vi "Add.vi"(8 "error in":errorcluster, 9 "configuration version":cluster{"major":u32, "minor":u32, "fix":u32}={"major"=1, "minor"=0, "fix"=0}, 10 "framework configuration":T1, 11 "target in":refnum<k24>) -> (0 "error out":errorcluster, 2 "data sharing framework custom device":T17 format="%.0x", 3 "target out":refnum<k24>)   [LabVIEW 2017, in "Data Sharing Framework Custom Device Scripting.lvlib"]
uses:
  Data Sharing Framework Custom Device Scripting.lvlib
  NationalInstruments.VeriStand.SystemDefinitionAPI
  <vilib>/NI Veristand/Custom Device API/Custom Device Item Ref.ctl
  DSF Core.lvlibp/Typedefs/DSF Engine Framework Configuration.ctl
  DSF Core.lvlibp/Typedefs/DSF Engine Plugin Configuration.ctl
  DSF Core.lvlibp/Typedefs/Core Plugin Configuration.ctl
  DSF Core.lvlibp/Typedefs/DSF Timing Info.ctl
  DSF Core.lvlibp/Typedefs/DSF Settings Info.ctl
  DSF Core.lvlibp/Typedefs/DSF Engine Plugin Thread Configuration.ctl
  DSF Core.lvlibp/Typedefs/Core Thread Configuration.ctl
  DSF Core.lvlibp/Typedefs/DSF Engine Transfer Group Configuration.ctl
  DSF Core.lvlibp/Typedefs/Core Group Configuration.ctl
  DSF Core.lvlibp/Typedefs/DSF Direction.ctl
  DSF Core.lvlibp/Typedefs/DSF Timeout Behavior.ctl
  DSF Core.lvlibp/Typedefs/DSF Engine Transfer Configuration.ctl
  DSF Core.lvlibp/Typedefs/Core Transfer Configuration.ctl
  DSF Core.lvlibp/Typedefs/DSF Engine Channel Configuration.ctl
  DSF Core.lvlibp/Typedefs/Core Channel Configuration.ctl
  DSF Core.lvlibp/Typedefs/DSF Data Type.ctl
  Shared/DSF Shared.lvlib
  System Explorer/DSF System Explorer.lvlib
  <vilib>/NI VeriStand/Custom Device API/Custom Device API.lvlib
  DSF Core.lvlibp
  DSF Core.lvlibp/Classes/Configuration/Core/Plugin/Plugin Configuration.lvclass
  DSF Core.lvlibp/Classes/Configuration/Core/Thread/Thread Configuration.lvclass
  DSF Core.lvlibp/Classes/Configuration/Core/Group/Group Configuration.lvclass
  DSF Core.lvlibp/Classes/Configuration/Core/Transfer/Transfer Configuration.lvclass
  DSF Core.lvlibp/Classes/Configuration/Core/Channel/Channel Configuration.lvclass
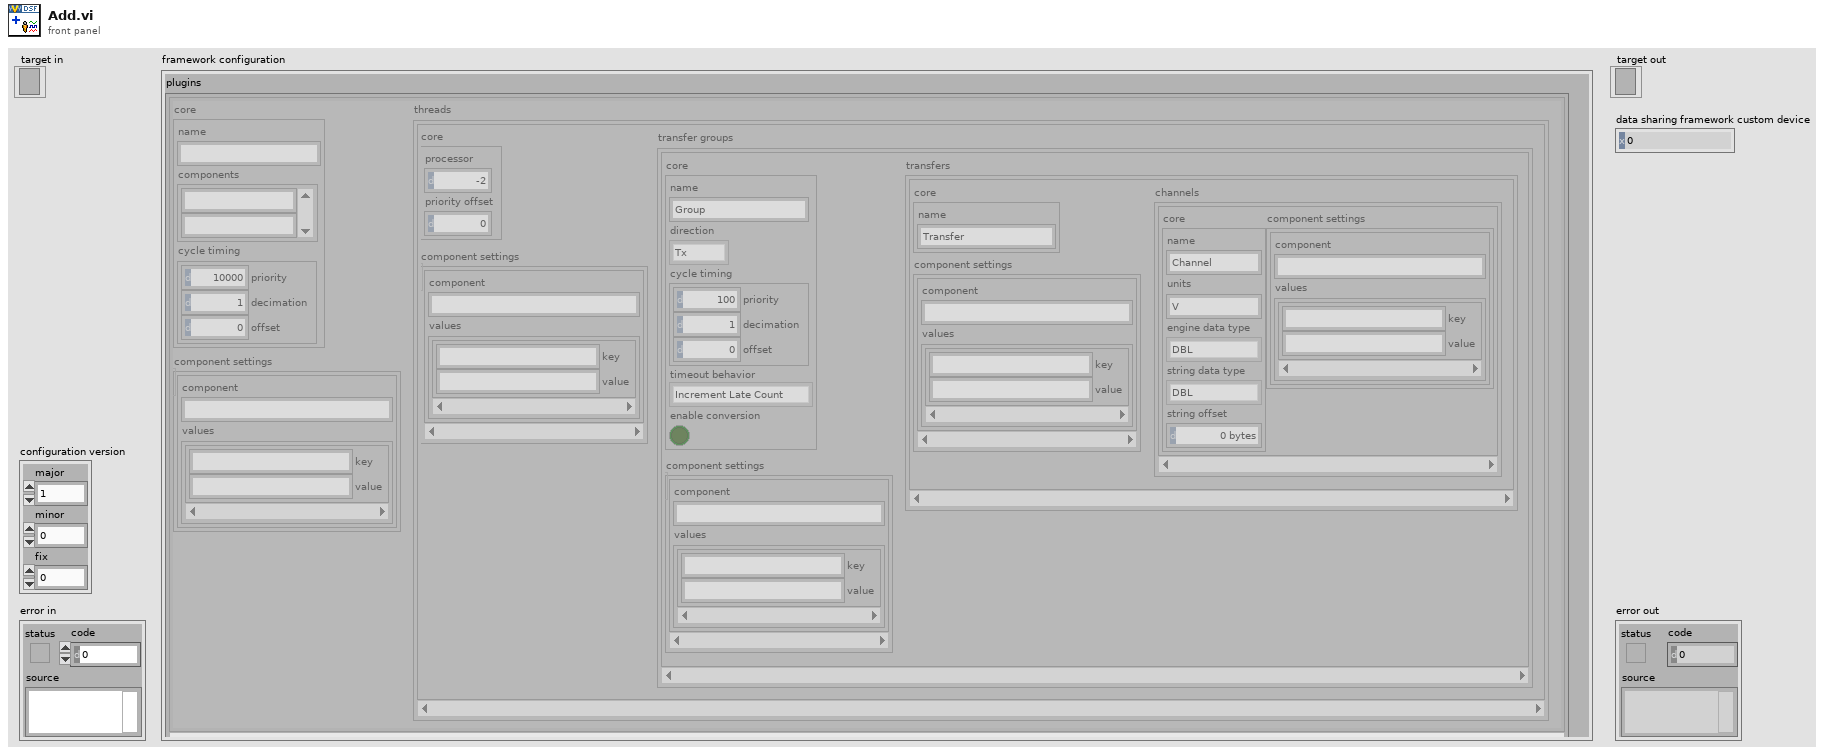
[diagram p1: front panel]
types:
  T1 = typedef "DSF Core.lvlibp/DSF Engine Framework Configuration.ctl" = cluster{"plugins":T2[]}
  T2 = typedef "DSF Core.lvlibp/DSF Engine Plugin Configuration.ctl" = cluster{"core":T3, "component settings":T5[], "threads":T6[]}
  T3 = typedef "DSF Core.lvlibp/Plugin Configuration.lvclass/Core Plugin Configuration.ctl" = cluster{"name":string, "components":string[], "cycle timing":T4}
  T4 = typedef "DSF Core.lvlibp/DSF Timing Info.ctl" = cluster{"priority":u64, "decimation":u64, "offset":u64}
  T5 = typedef "DSF Core.lvlibp/DSF Settings Info.ctl" = cluster{"component":string, "values":cluster{"key":string, "value":string}[]}
  T6 = typedef "DSF Core.lvlibp/DSF Engine Plugin Thread Configuration.ctl" = cluster{"core":T7, "component settings":T5[], "transfer groups":T8[]}
  T7 = typedef "DSF Core.lvlibp/Thread Configuration.lvclass/Core Thread Configuration.ctl" = cluster{"processor":i32, "priority offset":i16}
  T8 = typedef "DSF Core.lvlibp/DSF Engine Transfer Group Configuration.ctl" = cluster{"core":T9, "component settings":T5[], "transfers":T12[]}
  T9 = typedef "DSF Core.lvlibp/Group Configuration.lvclass/Core Group Configuration.ctl" = cluster{"name":string, "direction":T10, "cycle timing":T4, "timeout behavior":T11, "enable conversion":bool}
  T10 = typedef "DSF Core.lvlibp/DSF Direction.ctl" = enum8{"Tx", "Rx"}
  T11 = typedef "DSF Core.lvlibp/DSF Timeout Behavior.ctl" = enum8{"Increment Late Count", "Throw Error"}
  T12 = typedef "DSF Core.lvlibp/DSF Engine Transfer Configuration.ctl" = cluster{"core":T13, "component settings":T5[], "channels":T14[]}
  T13 = typedef "DSF Core.lvlibp/Transfer Configuration.lvclass/Core Transfer Configuration.ctl" = cluster{"name":string}
  T14 = typedef "DSF Core.lvlibp/DSF Engine Channel Configuration.ctl" = cluster{"core":T15, "component settings":T5[]}
  T15 = typedef "DSF Core.lvlibp/Channel Configuration.lvclass/Core Channel Configuration.ctl" = cluster{"name":string, "units":string, "engine data type":T16, "string data type":T16, "string offset":u64}
  T16 = typedef "DSF Core.lvlibp/DSF Data Type.ctl" = enum8{"Bool", "SGL", "DBL", "I8", "I16", "I32", "I64", "U8", "U16", "U32", "U64"}
  T17 = typedef "Custom Device API.lvlib/Custom Device Item Ref.ctl" = u64
  T18 = typedef "DSF Core.lvlibp/DSF Version Info.ctl" = cluster{"major":u32, "minor":u32, "fix":u32, "build":string}
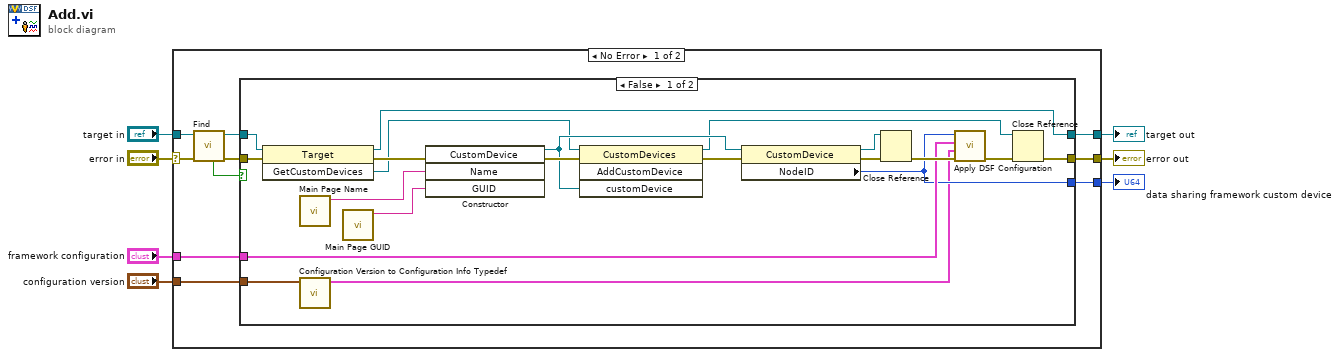
[diagram p0: block diagram]
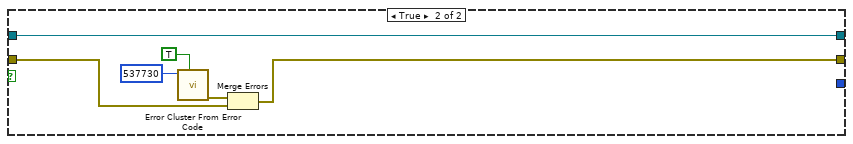
[diagram p2: hidden frame]
diagram:
  n1 = case shown="No Error" "error in" {
    selector: "error in" -> [w15 w45]
    tunnel: [w11 w45] -> w7
    tunnel: "target in" -> [w16 w44]
    tunnel: [w12 w44] -> w4
    tunnel: [w17 _] -> w3
    tunnel: "framework configuration" -> [w10 _]
    tunnel: "configuration version" -> [w9 _]
    frame No Error {
      n2 = call "Find.vi"("error in"=w15, "target in"=w16) -> ("error out"=w13:errorcluster, "target out"=w14:refnum<k24>, "found?"=w8:bool)  [unwired: 6 in, 1 out]
      n3 = case shown="False" w8 {
        tunnel: [w24 w41] -> w11
        tunnel: [w20 _] -> w17
        tunnel: w14 -> [w30 w39]
        tunnel: w13 -> [w29 w40]
        tunnel: [w28 w39] -> w12
        tunnel: w10 -> [w21 _]
        tunnel: w9 -> [w19 _]
        frame False {
          n4 = invoke class="Target" method="GetCustomDevices"(reference=w30, error in=w29) -> (reference out=w28:refnum<k24>, error out=w27:errorcluster, "GetCustomDevices"=w26:refnum<k24>)  [unwired: 1 in]
          n5 = call "Main Page Name.vi"() -> ("name"=w33:string)  [unwired: 11 in]
          n6 = call "Configuration Version to Configuration Info Typedef.vi"("configuration version"=w19) -> ("version info"=w18:T18)  [unwired: 10 in]
          n7 = call "Main Page GUID.vi"() -> ("Main Page GUID"=w31:string)  [unwired: 11 in]
          n8 = constructor class="CustomDevice"(error in=w27, "Name"=w33, "GUID"=w31) -> (reference out=w32:refnum<k24>, error out=w37:errorcluster)  [unwired: 2 in, 3 out]
          n9 = invoke class="CustomDevices" method="AddCustomDevice"(reference=w26, error in=w37, "customDevice"=w32) -> (reference out=w25:refnum<k24>, error out=w36:errorcluster)  [unwired: 1 in, 2 out]
          n10 = property class="CustomDevice"(reference=w32, error in=w36) -> (reference out=w35:refnum<k24>, error out=w34:errorcluster, "NodeID"=w20:u64)
          n11 = Close Reference(reference=w35, error in (no error)=w34) -> (error out=w23:errorcluster)
          n12 = call "Apply DSF Configuration.vi"("error in (no error)"=w23, "version"=w18, "framework configuration"=w21, "Item Ref in"=w20) -> ("error out"=w22:errorcluster)  [unwired: 7 in]
          n13 = Close Reference(reference=w25, error in (no error)=w22) -> (error out=w24:errorcluster)
        }
        frame True {
          n14 = call <vilib>:"Error Cluster From Error Code.vi"("show call chain? (False)"=TRUE, "error code (0)"=537730) -> ("error out"=w42:errorcluster)  [unwired: 7 in]
          n15 = Merge Errors(w42, w40) -> (w41:errorcluster)
        }
      }
    }
    frame Error {
    }
  }
  "target out" <- w4
  "error out" <- w7
  "data sharing framework custom device" <- w3
